vi "Initialize.vi"(8 "Error In":errorcluster, 11 "MainData":T1) -> (0 "Error Out":errorcluster, 3 "MainData out":T1)   [LabVIEW 2019, in "MainController.lvlib"]
uses:
  MainController.lvlib
  Cluster - MainData.ctl
  All Message Queues.ctl
  Cluster - MainControllerMessage.ctl
  Enum - MainState.ctl
  AutoMode/Cluster - AutoModeMessage.ctl
  AutoMode/Enum - AutoModeState.ctl
  ManualMode/Cluster - ManualModeMessageCluster.ctl
  ManualMode/Enum - ManualModeMessage.ctl
  Settings/CTL_MessageCluster.ctl
  Settings/CTL_SettingsMessage.ctl
  Cluster - HardwareConfiguration.ctl
  Cluster - LoggingConfiguration.ctl
  Cluster - TestSettings.ctl
  UI State.ctl
  UI Data.ctl
  Settings/Cluster - Settings.ctl
  Settings/Settings.lvlib
  AutoMode/AutoMode.lvlib
  ManualMode/ManualMode.lvlib
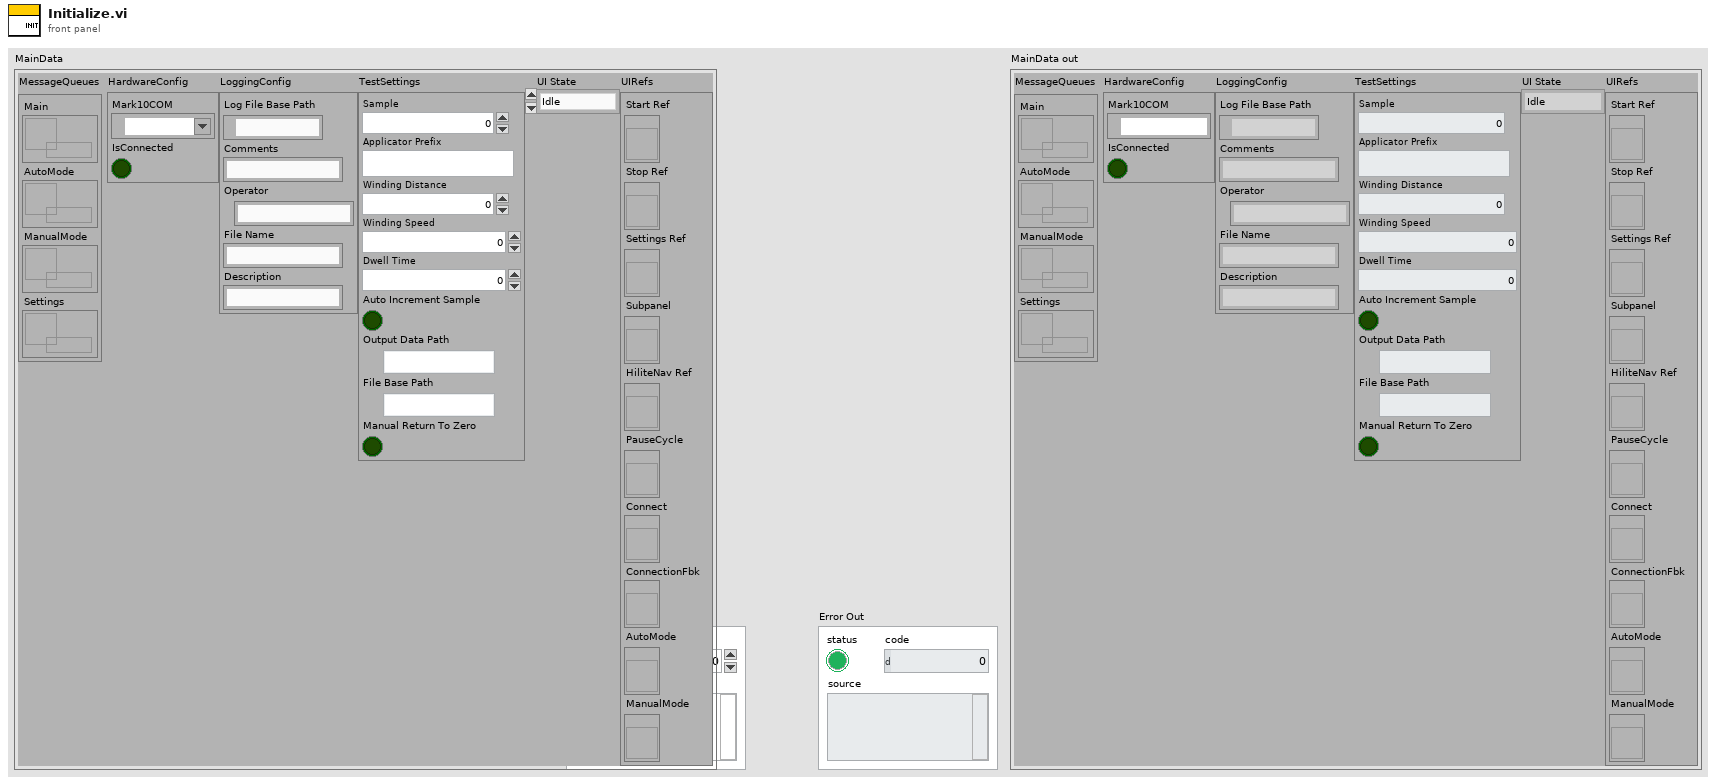
[diagram p1: front panel]
types:
  T1 = typedef "MainController.lvlib/Cluster - MainData.ctl" = cluster{"MessageQueues":T2, "HardwareConfig":T3, "LoggingConfig":T4, "TestSettings":T5, "UI State":T6, "UIRefs":T7}
  T2 = typedef "MainController.lvlib/All Message Queues.ctl" = cluster{"Main":refnum<queue>, "AutoMode":refnum<queue>, "ManualMode":refnum<queue>, "Settings":refnum<queue>}
  T3 = typedef "MainController.lvlib/Cluster - HardwareConfiguration.ctl" = cluster{"Mark10COM":refnum<visa-resource-name>, "IsConnected":bool}
  T4 = typedef "MainController.lvlib/Cluster - LoggingConfiguration.ctl" = cluster{"Log File Base Path":path, "Comments ":string, "Operator":string, "File Name":string, "Description":string}
  T5 = typedef "MainController.lvlib/Cluster - TestSettings.ctl" = cluster{"Sample":u32, "Applicator Prefix":string, "Winding Distance":dbl, "Winding Speed":dbl, "Dwell Time":dbl, "Auto Increment Sample":bool, "Output Data Path":path, "File Base Path":path, "Manual Return To Zero":bool}
  T6 = typedef "MainController.lvlib/UI State.ctl" = enum16{"Idle", "AutoIdle", "AutoRunning", "ManualMode", "Settings"}
  T7 = typedef "MainController.lvlib/UI Data.ctl" = cluster{"Start Ref":refnum<vi>, "Stop Ref":refnum<vi>, "Settings Ref":refnum<vi>, "Subpanel":refnum<vi>, "HiliteNav Ref":refnum<vi>, "PauseCycle":refnum<vi>, "Connect":refnum<vi>, "ConnectionFbk":refnum<vi>, "AutoMode":refnum<vi>, "ManualMode":refnum<vi>}
  T8 = typedef "Settings.lvlib/Cluster - Settings.ctl" = cluster{"Hardware Configuration":T3, "TestSettings":T5}
  T9 = typedef "MainController.lvlib/Enum - MainState.ctl" = enum16{"Initialize", "InitUIRefs", "LaunchSettings", "LaunchAutoMode", "LaunchManualMode", "LaunchTestReport", "ConnectHardware", "DisconnectHardware", "HiliteNavItems", "StartAutoMode", "PauseAutoMode", "StopAutoMode", "ShowFlyout", "HideFlyout", "BroadcastSettings", "PickupTestSettings", "BroadcastHW", "AutoTestDone", "DAQStatus", "UpdateCommandBar", "Error", "RecieveError", "Exit"}
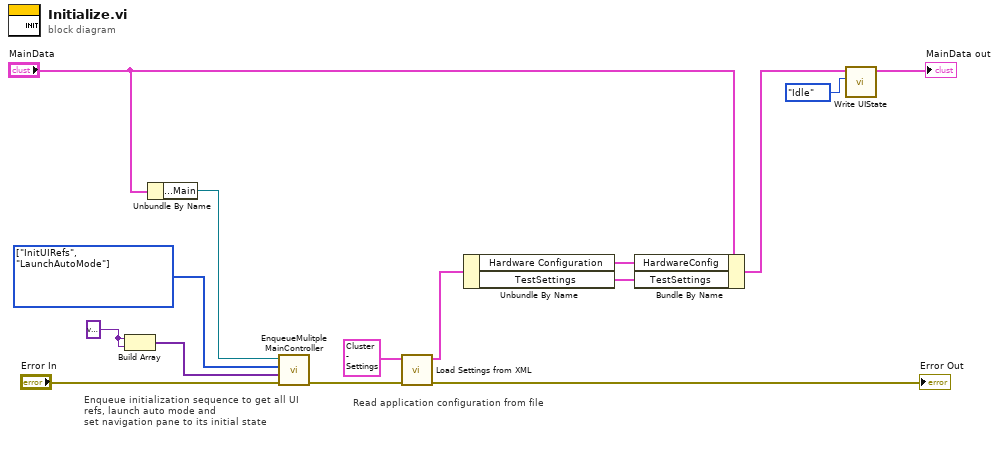
[diagram p0: block diagram]
diagram:
  w13 = variant
  w14 = T9[] [enum."InitUIRefs", enum."LaunchAutoMode"] items=["Initialize", "InitUIRefs", "LaunchSettings", "LaunchAutoMode", "LaunchManualMode", "LaunchTestReport", "ConnectHardware", "DisconnectHardware", "HiliteNavItems", "StartAutoMode", "PauseAutoMode", "StopAutoMode", "ShowFlyout", "HideFlyout", "BroadcastSettings", "PickupTestSettings", "BroadcastHW", "AutoTestDone", "DAQStatus", "UpdateCommandBar", "Error", "RecieveError", "Exit"] ("Messages")
  # "Read application configuration from file"
  # "Enqueue initialization sequence to get all UI refs, launch auto mode and\nset navigation pane to its initial state"
  n1 = Build Array(w13, w13) -> (w12:variant[])
  n2 = Unbundle By Name("MainData") -> ("MessageQueues.Main"=w15:refnum<queue>)
  n3 = call "EnqueueMulitpleMainController.vi"("error in (no error)"="Error In", "Data"=w12, "Messages"=w14, "MainQueue"=w15) -> ("error out"=w11:errorcluster)  [unwired: 5 in, 2 out]
  n4 = call "Load Settings from XML.vi"("error in (no error)"=w11, "Settings"=T8 {"Hardware Configuration"={"Mark10COM"="", "IsConnected"=FALSE}, "TestSettings"={"Sample"=0, "Applicator Prefix"="", "Winding Distance"=0.0, "Winding Speed"=0.0, "Dwell Time"=0.0, "Auto Increment Sample"=FALSE, "Output Data Path"=path "", "File Base Path"=path "", "Manual Return To Zero"=FALSE}}) -> ("error out"=→"Error Out":errorcluster, "Settings out"=w10:T8)  [unwired: 8 in]
  n5 = Unbundle By Name(w10) -> ("Hardware Configuration"=w9:T3, "TestSettings"=w8:T5)
  n6 = Bundle By Name(cluster="MainData", "HardwareConfig"=w9, "TestSettings"=w8) -> (w4:T1)
  n7 = call "Write UIState.vi"("UI State"=UI_State."Idle", "MainData"=w4) -> ("MainData out"=→"MainData out":T1)  [unwired: 9 in]
